vi "parse.onsaleDate.vi"(0 "dates":cluster{"type":string, "date":string}[](array[cluster])) -> (1 "Time Stamp":timestamp, 2 "date string":string)   [LabVIEW 2024]
uses:
  <vilib>/addons/_JKI.lib/Serialization/JSON/Deserializer/JSON Deserializer/JSON Deserializer.lvclass
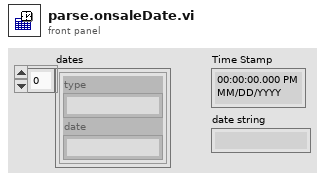
[diagram p1: front panel]
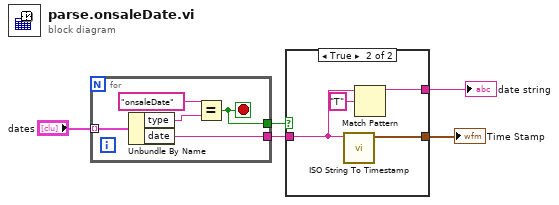
[diagram p0: block diagram]
diagram:
  n1 = for {
    tunnel: "dates" -> [w10] mode=indexing
    tunnel: [w7] -> w3
    tunnel: [w6] -> w1
    stop <- w6 stop-if-true
    n2 = Unbundle By Name(w10) -> ("type"=w9:string, "date"=w7:string)
    n3 = Equal?(x="onsaleDate", y=w9) -> (x = y?=w6:bool)
  }
  n4 = case shown="True" w1 {
    tunnel: [_ w14] -> w4
    tunnel: w3 -> [_ w13]
    tunnel: [_ w11] -> w2
    frame False {
    }
    frame True {
      n5 = call <vilib>:"ISO String To Timestamp.vi"("ISO Timestamp String"=w13) -> ("Time Stamp"=w14:timestamp)  [unwired: 9 in, 1 out]
      n6 = Match Pattern(string=w13, regular expression="T") -> (before substring=w11:string)  [unwired: 1 in, 3 out]
    }
  }
  "Time Stamp" <- w4
  "date string" <- w2
